vi "BRig_RT__Case_Exp__storeData__endExp__v5__p1__wait.vi"(0 "input_dataCurrent":u16[](array[numeric]), 1 "input_dataLC":u16[](array[numeric]), 2 "input_dataExp":u16[](array[numeric]), 5 "input_dataBlock":u16[][](array[numeric]), 9 "input_dataExp_end":u16[](array[numeric]), 11 "input_dataLC_end":u16[](array[numeric])) -> (8 "output_True":bool)   [LabVIEW 2014]
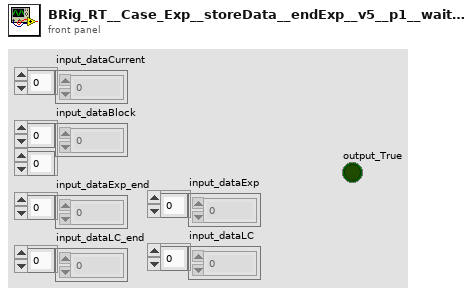
[diagram p1: front panel]
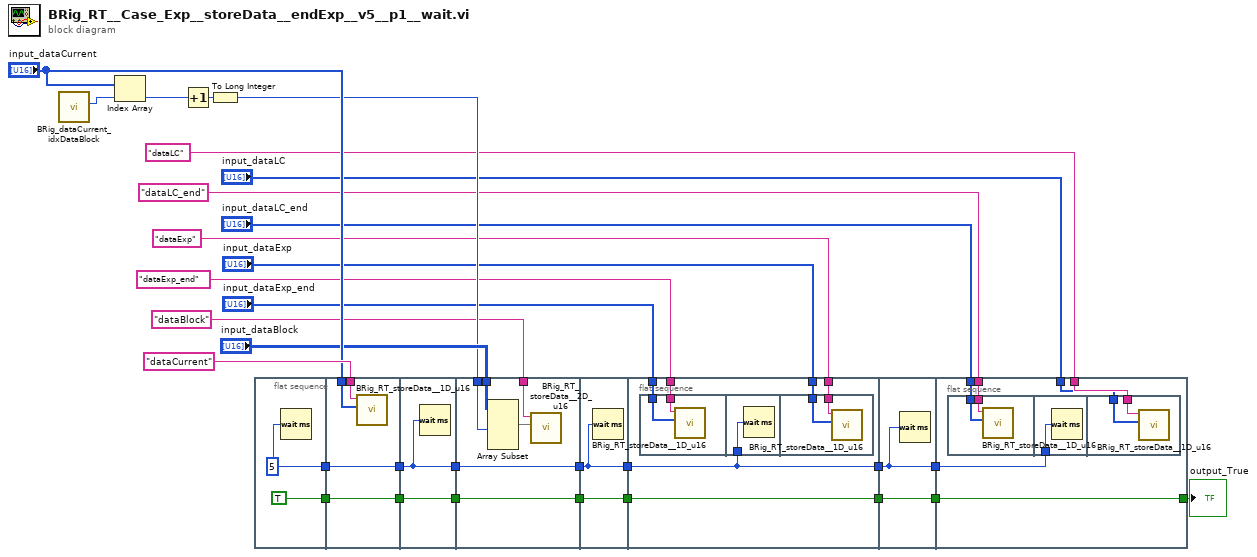
[diagram p0: block diagram]
diagram:
  n1 = call "BRig_dataCurrent_idxDataBlock.vi"() -> ("output_idxDataBlock"=w18:i32)  [unwired: 11 in]
  n2 = Index Array(array="input_dataCurrent", index=w18) -> (element=w17:u16)
  n3 = Increment(x=w17) -> (x+1=w16:u16)
  n4 = To Long Integer(number=w16) -> (32bit integer=w28:i32)
  n5 = flat-sequence {
    tunnel: [TRUE] -> w14
    tunnel: [w32] -> w7
    tunnel: "dataCurrent" ("input_filename") -> [w37]
    tunnel: "input_dataCurrent" -> [w36]
    tunnel: [w35] -> w13
    tunnel: w14 -> [w35]
    tunnel: w7 -> [w34]
    tunnel: [w34] -> w6
    tunnel: w13 -> [w39]
    tunnel: [w39] -> w12
    tunnel: w6 -> [w38]
    tunnel: [w38] -> w5
    tunnel: "input_dataBlock" -> [w45]
    tunnel: w28 -> [w44]
    tunnel: "dataBlock" ("input_filename") -> [w42]
    tunnel: [w41] -> w11
    tunnel: w12 -> [w41]
    tunnel: w5 -> [w40]
    tunnel: [w40] -> w4
    tunnel: w11 -> [w47]
    tunnel: [w47] -> w10
    tunnel: w4 -> [w46]
    tunnel: [w46] -> w3
    tunnel: "input_dataExp_end" -> [w53]
    tunnel: "dataExp_end" ("input_filename") -> [w52]
    tunnel: "input_dataExp" -> [w51]
    tunnel: "dataExp" ("input_filename") -> [w50]
    tunnel: [w49] -> w9
    tunnel: w10 -> [w49]
    tunnel: w3 -> [w48]
    tunnel: [w48] -> w2
    tunnel: w9 -> [w60]
    tunnel: [w60] -> w8
    tunnel: w2 -> [w59]
    tunnel: [w59] -> w1
    tunnel: "input_dataLC_end" -> [w66]
    tunnel: "dataLC_end" ("input_filename") -> [w65]
    tunnel: "dataLC" ("input_filename") -> [w64]
    tunnel: "input_dataLC" -> [w63]
    tunnel: w8 -> [w62]
    tunnel: [w62] -> w15
    tunnel: w1 -> [w61]
    frame #0 {
      w32 = u32 5 ("milliseconds to wait")
      n6 = Wait (ms)(milliseconds to wait=w32) -> ()  [unwired: 1 out]
    }
    frame #1 {
      n7 = call "BRig_RT_storeData__1D_u16.vi"("Array"=w36, "input_filename"=w37) -> ()  [unwired: 10 in]
    }
    frame #2 {
      n8 = Wait (ms)(milliseconds to wait=w38) -> ()  [unwired: 1 out]
    }
    frame #3 {
      n9 = Array Subset(array=w45, length (row)=w44) -> (w43:u16[][])  [unwired: 3 in]
      n10 = call "BRig_RT_storeData__2D_u16.vi"("Array"=w43, "input_filename"=w42) -> ()  [unwired: 10 in]
    }
    frame #4 {
      n11 = Wait (ms)(milliseconds to wait=w46) -> ()  [unwired: 1 out]
    }
    frame #5 {
      n12 = flat-sequence {
        tunnel: w53 -> [w55]
        tunnel: w52 -> [w54]
        tunnel: w48 -> [w56]
        tunnel: w51 -> [w57]
        tunnel: w50 -> [w58]
        frame #0 {
          n13 = call "BRig_RT_storeData__1D_u16.vi"("Array"=w55, "input_filename"=w54) -> ()  [unwired: 10 in]
        }
        frame #1 {
          n14 = Wait (ms)(milliseconds to wait=w56) -> ()  [unwired: 1 out]
        }
        frame #2 {
          n15 = call "BRig_RT_storeData__1D_u16.vi"("Array"=w57, "input_filename"=w58) -> ()  [unwired: 10 in]
        }
      }
    }
    frame #6 {
      n16 = Wait (ms)(milliseconds to wait=w59) -> ()  [unwired: 1 out]
    }
    frame #7 {
      n17 = flat-sequence {
        tunnel: w66 -> [w68]
        tunnel: w65 -> [w67]
        tunnel: w61 -> [w69]
        tunnel: w64 -> [w71]
        tunnel: w63 -> [w70]
        frame #0 {
          n18 = call "BRig_RT_storeData__1D_u16.vi"("Array"=w68, "input_filename"=w67) -> ()  [unwired: 10 in]
        }
        frame #1 {
          n19 = Wait (ms)(milliseconds to wait=w69) -> ()  [unwired: 1 out]
        }
        frame #2 {
          n20 = call "BRig_RT_storeData__1D_u16.vi"("Array"=w70, "input_filename"=w71) -> ()  [unwired: 10 in]
        }
      }
    }
  }
  "output_True" <- w15
